vi "DateTime (Read).vi"(6 "ISOBUS address":T2=-1 caption="ISOBUS address (-1)", 8 "error in":errorcluster, 11 "Mercury Reference In":T3) -> (0 "error out":errorcluster, 2 "time stamp":timestamp, 3 "Mercury Reference Out":T3, 4 "Valid?":T1)   [LabVIEW 2015, in "Mercury iXX.lvlib" / "System.lvlib"]
doc: "Returns the current instrument date and time."
uses:
  System.lvlib
  Controls/Mercury Reference.ctl
  Controls/Comms Transport Layer.ctl
  private/Controls/Query Dynamic Reference.ctl
  Controls/ISOBus Address.ctl
  Controls/Is Valid LED.ctl
  <vilib>/Utility/miscctls.llb/LVDateTimeRec.ctl
  Mercury iXX.lvlib
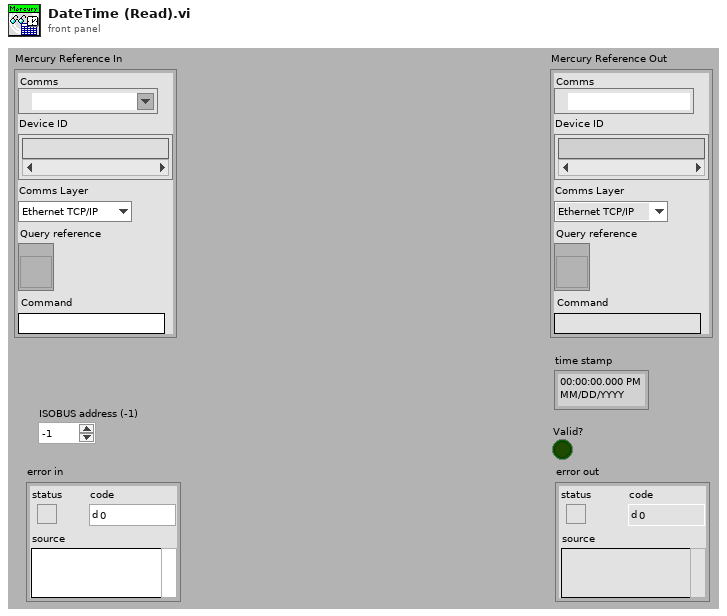
[diagram p1: front panel]
types:
  T1 = typedef "Mercury iXX.lvlib/Is Valid LED.ctl" = bool
  T2 = typedef "Mercury iXX.lvlib/ISOBus Address.ctl" = i32
  T3 = typedef "Mercury iXX.lvlib/Mercury Reference.ctl" = cluster{"Comms":refnum<visa-resource-name>, "Device ID":string[], "Comms Layer":T4, "Command":string, "Query reference":T5}
  T4 = typedef "Mercury iXX.lvlib/Comms Transport Layer.ctl" = enum16{"Ethernet TCP/IP", "USB", "ISOBus - RS-232", "GPIB"}
  T5 = typedef "Mercury iXX.lvlib/Query Dynamic Reference.ctl" = refnum<vi>
  T6 = typedef "LVDateTimeRec.ctl" = cluster{"fractional second":dbl, "second":i32, "minute":i32, "hour":i32, "day of month":i32, "month":i32, "year":i32, "day of week":i32, "day of year":i32, "DST":i32}
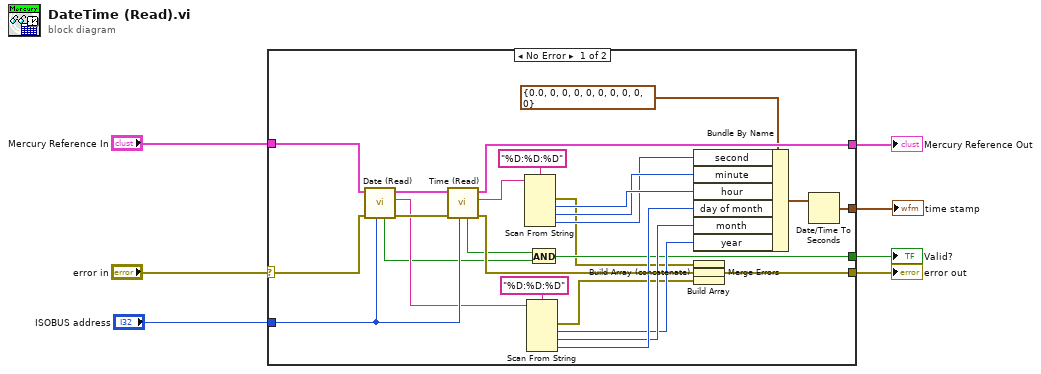
[diagram p0: block diagram]
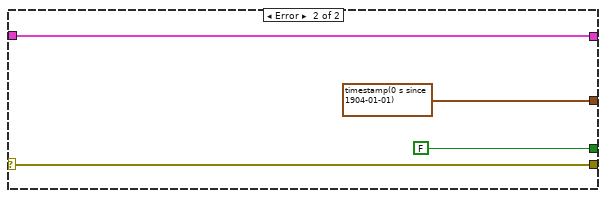
[diagram p2: hidden frame]
diagram:
  n1 = case shown="No Error" "error in" {
    selector: "error in" -> [w34 w38]
    tunnel: "Mercury Reference In" -> [w35 w39]
    tunnel: [w29 w39] -> w6
    tunnel: [w12 w38] -> w5
    tunnel: "ISOBUS address" -> [w31 _]
    tunnel: [w28 timestamp(0 s since 1904-01-01) ("time stamp")] -> w2
    tunnel: [w15 FALSE] -> w1
    frame No Error {
      n2 = call "Date (Read).vi"("ISOBUS address"=w31, "error in"=w34, "Mercury Reference In"=w35) -> ("error out"=w32:errorcluster, "Date"=w19:string, "Mercury Reference Out"=w33:T3, "Valid?"=w14:T1)  [unwired: 1 in, 4 out]
      n3 = call "Time (Read).vi"("ISOBUS address"=w31, "error in"=w32, "Mercury Reference In"=w33) -> ("error out"=w30:errorcluster, "Time"=w25:string, "Mercury Reference Out"=w29:T3, "Valid?"=w13:T1)  [unwired: 5 out]
      n4 = Scan From String(format string="%D:%D:%D", input string=w25) -> (error out=w11:errorcluster, output 1=w23:i32, output 2=w22:i32, output 3=w21:i32)  [unwired: 2 in, 5 out]
      n5 = Scan From String(format string="%D:%D:%D", input string=w19) -> (error out=w10:errorcluster, output 1=w16:i32, output 2=w17:i32, output 3=w18:i32)  [unwired: 2 in, 5 out]
      n6 = And(x=w13, y=w14) -> (x .and. y?=w15:T1)
      n7 = Bundle By Name(cluster=T6 {"fractional second"=0.0, "second"=0, "minute"=0, "hour"=0, "day of month"=0, "month"=0, "year"=0, "day of week"=0, "day of year"=0, "DST"=0} ("date time rec"), "second"=w21, "minute"=w22, "hour"=w23, "day of month"=w18, "month"=w17, "year"=w16) -> (w26:T6)
      n8 = Build Array(w11, w30, w10) -> (w9:errorcluster[])
      n9 = Build Array (concatenate)(w9) -> (w8:errorcluster[])
      n10 = Merge Errors(w8) -> (w12:errorcluster)
      n11 = Date/Time To Seconds(2:w26) -> (0:w28:timestamp)  [unwired: 1 out]
    }
    frame Error {
    }
  }
  "Mercury Reference Out" <- w6
  "error out" <- w5
  "time stamp" <- w2
  "Valid?" <- w1
